vi "Day 7-1.vi"() -> ()   [LabVIEW 2019, in "Day 7.lvlib"]
uses:
  Day 7.lvlib
  <vilib>/Analysis/NI_AALBase.lvlib
panel:
  out "sum":i32
  out "median":i32
  out "array":i32[](array[numeric])
  in  "String":string
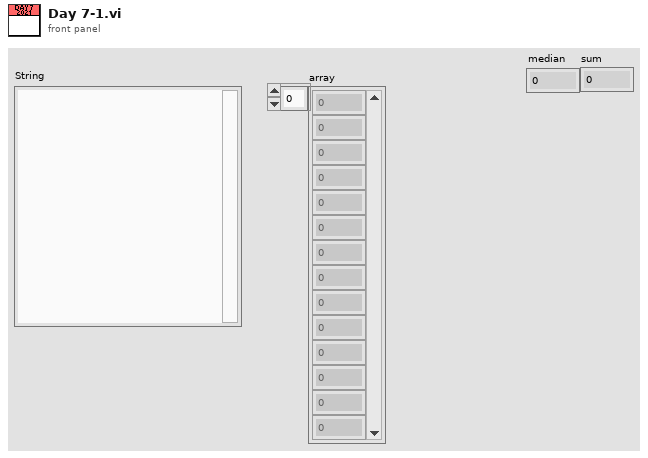
[diagram p1: front panel]
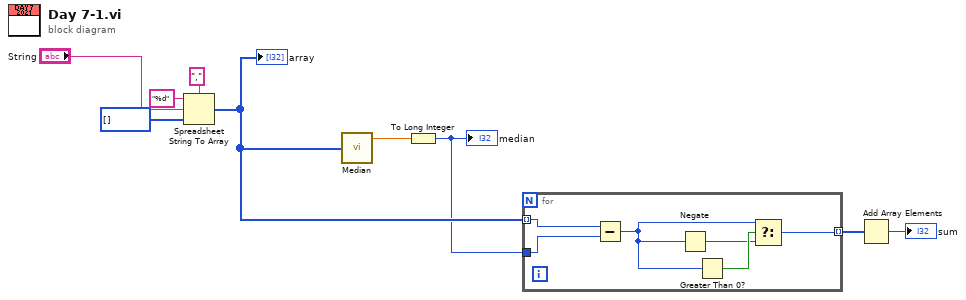
[diagram p0: block diagram]
diagram:
  n1 = Spreadsheet String To Array(delimiter (Tab)=",", format string="%d", spreadsheet string="String", array type (2D Dbl)=i32[] []) -> (array=w4:i32[])
  "array" <- w4
  n2 = call <vilib>:"Median.vi"("X"=w4) -> ("median"=w5:dbl)  [unwired: 1 out]
  n3 = To Long Integer(number=w5) -> (32bit integer=w3:i32)
  "median" <- w3
  n4 = for {
    tunnel: w4 -> [w15] mode=indexing
    tunnel: w3 -> [w14]
    tunnel: [w10] -> w2 mode=indexing
    n5 = Subtract(x=w15, y=w14) -> (x-y=w12:i32)
    n6 = Negate(x=w12) -> (-x=w11:i32)
    n7 = Greater Than 0?(x=w12) -> (x > 0?=w13:bool)
    n8 = Select(t=w12, s=w13, f=w11) -> (s? t:f=w10:i32)
  }
  n9 = Add Array Elements(numeric array=w2) -> (sum=→"sum":i32)
